vi "Assert String Contains String.vi"(5 "Needle":string, 7 "Message (\"\")":string, 8 "error in (no error)":errorcluster, 10 "Haystack":string) -> (0 "error out":errorcluster)   [LabVIEW 2017, in "Assertion.lvlib"]
doc: "Asserts that <B>haystack</B> contains <B>needle</B>. Does nothing if an error occurred before this node runs. Returns an error if the assertion failed. Optionally adds a message to the error message if the assertion failed."
uses:
  Assertion.lvlib
  Constraint/StringContains/StringContains.lvclass
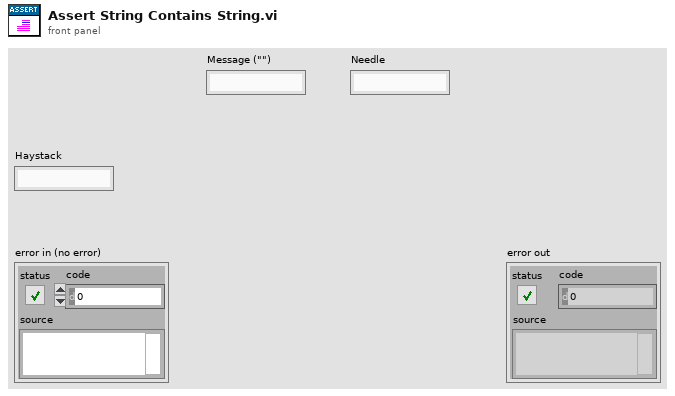
[diagram p1: front panel]
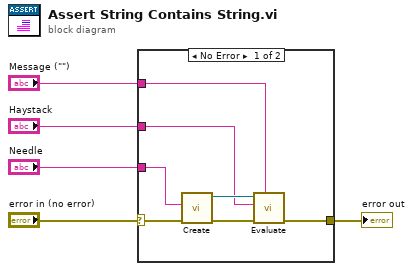
[diagram p0: block diagram]
diagram:
  n1 = case shown="No Error" "error in (no error)" {
    selector: "error in (no error)" -> [w7 w13]
    tunnel: "Haystack" -> [w10 _]
    tunnel: [w9 w13] -> w4
    tunnel: "Message (\"\")" -> [w8 _]
    tunnel: "Needle" -> [w6 _]
    frame No Error {
      n2 = call "Create.vi"("error in (no error)"=w7, "Needle"=w6) -> ("error out"=w11:errorcluster, "StringContains"=w12:refnum<class "StringContains.lvclass">)  [unwired: 8 in]
      n3 = call-dynamic "Evaluate.vi"("Message (\"\")"=w8, "error in (no error)"=w11, "Actual"=w10, "Constraint in"=w12) -> ("error out"=w9:errorcluster)  [unwired: 6 in, 1 out]
    }
    frame Error {
    }
  }
  "error out" <- w4
